vi "Bounds.vi"(1 "XRef":refnum<vi>, 2 "State In":T2={"Enum Type"=variant(dbl 0.0), "Types Type"=variant, "Enum Names"=[], "Type Names"=[], "Typedef Name"="", "Typedef Path"=path ""}) -> (0 "Bounds":cluster{"Width":T1, "Height":T1})   [LabVIEW 2015, in "Define-Tagged-Union.xnode"]
doc: "This ability VI is used to tell LabVIEW your current bounds. If you want to update your bounds, you must inform LabVIEW through the UpdateImageAndBounds reply of another ability VI. If you change your bounds, you will also probably want to update your image.\n\nDefault behavior: None.\n\nThis ability does not provide UI and OS messages are not handled."
uses:
  Define-Tagged-Union.xnode
  State.ctl
  <vilib>/XNodeSupport/XNodeInt.ctl
  <vilib>/XNodeSupport/NI_XNodeSupport.lvlib
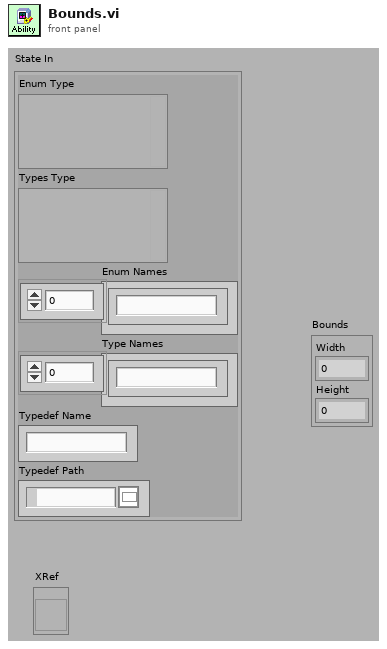
[diagram p1: front panel]
types:
  T1 = typedef "NI_XNodeSupport.lvlib/XNodeInt.ctl" = i32
  T2 = typedef "Define-Tagged-Union.xnode/State.ctl" = cluster{"Enum Type":variant, "Types Type":variant, "Enum Names":string[], "Type Names":string[], "Typedef Name":string, "Typedef Path":path}
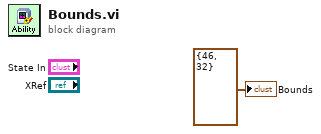
[diagram p0: block diagram]
diagram:
  "Bounds" <- cluster{"Width":T1, "Height":T1} {"Width"=46, "Height"=32} ("Bounds")
